vi "Model Calibration Control - 1D Table.vi"() -> ()   [LabVIEW 2011]
doc: "Sample numeric display item."
uses:
  <vilib>/NI Veristand/Display Template Support/Display Template Support.llb/cluster_Screen Item Settings.ctl
  <vilib>/NI Veristand/Display Template Support/Display Template Support.llb/cluster_Graph Scale Settings.ctl
  <vilib>/NI Veristand/Display Template Support/Display Template Support.llb/cluster_Graph Plot Settings.ctl
  NationalInstruments.VeriStand.SystemStorage
  Tables/TBL1D.xctl
  <vilib>/NI Veristand/Display Template Support/Display Template Support.llb/enum_Display Template Handler Minimal To Widget Msg.ctl
  <vilib>/NI Veristand/Display Template Support/Display Template Support.llb/enum_Display Template Handler Minimal To Workspace.ctl
  Tables/Limits TBL1D.ctl
  <vilib>/NI Veristand/Execution/Workspace/SystemState.ctl
  <vilib>/NI Veristand/Display Template Support/Display Template Support.llb/sub_Display Template Handler Custom.vi
  <vilib>/NI Veristand/Execution/ModelManager/NI VeriStand - Set Parameter 2D Array Values.vi
  <vilib>/NI Veristand/Execution/Workspace/NI VeriStand - Get Single Channel Value.vi
  <vilib>/NI Veristand/Execution/ModelManager/NI_VS ModelManager ExecutionAPI.lvlib
  <vilib>/NI Veristand/Execution/Workspace/NI_VS Workspace ExecutionAPI.lvlib
panel:
  in  "Paths":string[](array[string])
  out "Selected Parameter":string
  in  "TBL1D":cluster{"X":sgl[], "Y":sgl[]}(xcontrol)
  in  "NIVS.System Definition Root":refnum<k24>
  in  "Item.Data":T1
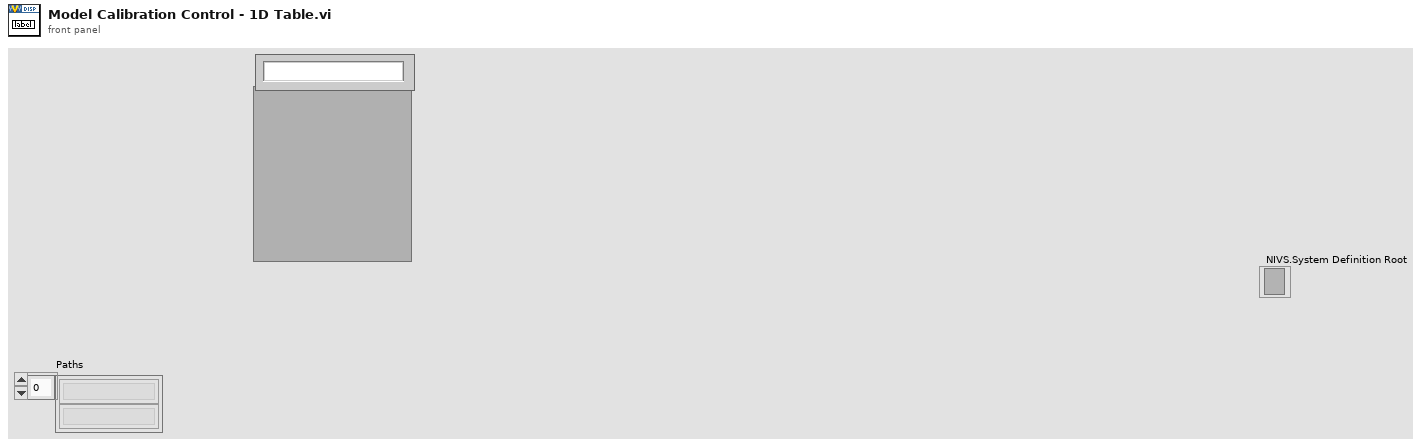
[diagram p1: front panel]
types:
  T1 = typedef "cluster_Screen Item Settings.ctl" = cluster{"Template VI":string, "Position X":i32, "Position Y":i32, "Custom":string, "Show Title Bar":bool, "ID":i32, "Always On Top":bool, "Allow Resize":bool, "Allow Minimize":bool, "Allow Close":bool, "Size to Screen":bool, "Screen.ID":i32, "State":enum16{"Normal", "New"}, "Title":string, "Window Bounds":cluster{"[0]":i16, "[1]":i16, "[2]":i16, "[3]":i16}, "Channel Ref":u64, "Unit":string, "Default Units?":bool, "Flash Limit?":bool, "Color 1":u32, "Color 2":u32, "Color 3":u32, "Color 4":u32, "Bck Color":u32, "Fore Color":u32, "Limit 1":dbl, "Limit 2":dbl, "Limit 3":dbl, "Limit 4":dbl, "Limit Mode 1":i32, "Limit Mode 2":i32, "Limit Mode 3":i32, "Limit Mode 4":i32, "Scale Precision":i32, "Scale Min":dbl, "Scale Max":dbl, "Format":i32, "Precision":i32, "Background Type":i32, "IDs":i32[], "Units":string[], "Labels":string[], "Scale Factor":dbl, "Scale Offset":dbl, "YScale Index":u32[], "XScale":T2, "YScales":T2[], "Plots":T3[], "Update Period":dbl, "History Length":dbl, "My.Ref":refnum<vi>, "Is Control?":bool, "Channel Paths":string[], "Custom Data":variant}
  T2 = typedef "cluster_Graph Scale Settings.ctl" = cluster{"Format":u8, "Precision":u8, "Fit":u8, "Label":string, "Use Default Label":bool, "Label Visible":bool, "Min":dbl, "Max":dbl}
  T3 = typedef "cluster_Graph Plot Settings.ctl" = cluster{"Bar Style":u8, "Fill To":i16, "Fill/PtColor":u32, "Line Style":u8, "Line Width":u8, "Color":u32, "Interp":u8, "Point Style":u8}
  T4 = typedef "TBL1D.xctl/Limits TBL1D.ctl" = cluster{"Min X":sgl, "Max X":sgl, "MaxDiff X":sgl, "MaxGrad X":sgl, "Min Y":sgl, "Max Y":sgl, "MaxDiff Y":sgl}
  T5 = typedef "enum_Display Template Handler Minimal To Workspace.ctl" = cluster{"Operation":enum16{"SetCustomData", "DeleteItem"}, "Data":variant}
  T6 = typedef "enum_Display Template Handler Minimal To Widget Msg.ctl" = enum16{"Stop", "LaunchConfigDialog"}
  T7 = typedef "NI_VS Workspace ExecutionAPI.lvlib/WorkspaceAPI.ctl" = refnum<k24>
  T8 = typedef "NI_VS ModelManager ExecutionAPI.lvlib/ModelManagerAPI.ctl" = refnum<k24>
  T9 = typedef "NI_VS Workspace ExecutionAPI.lvlib/SystemState.ctl" = u8
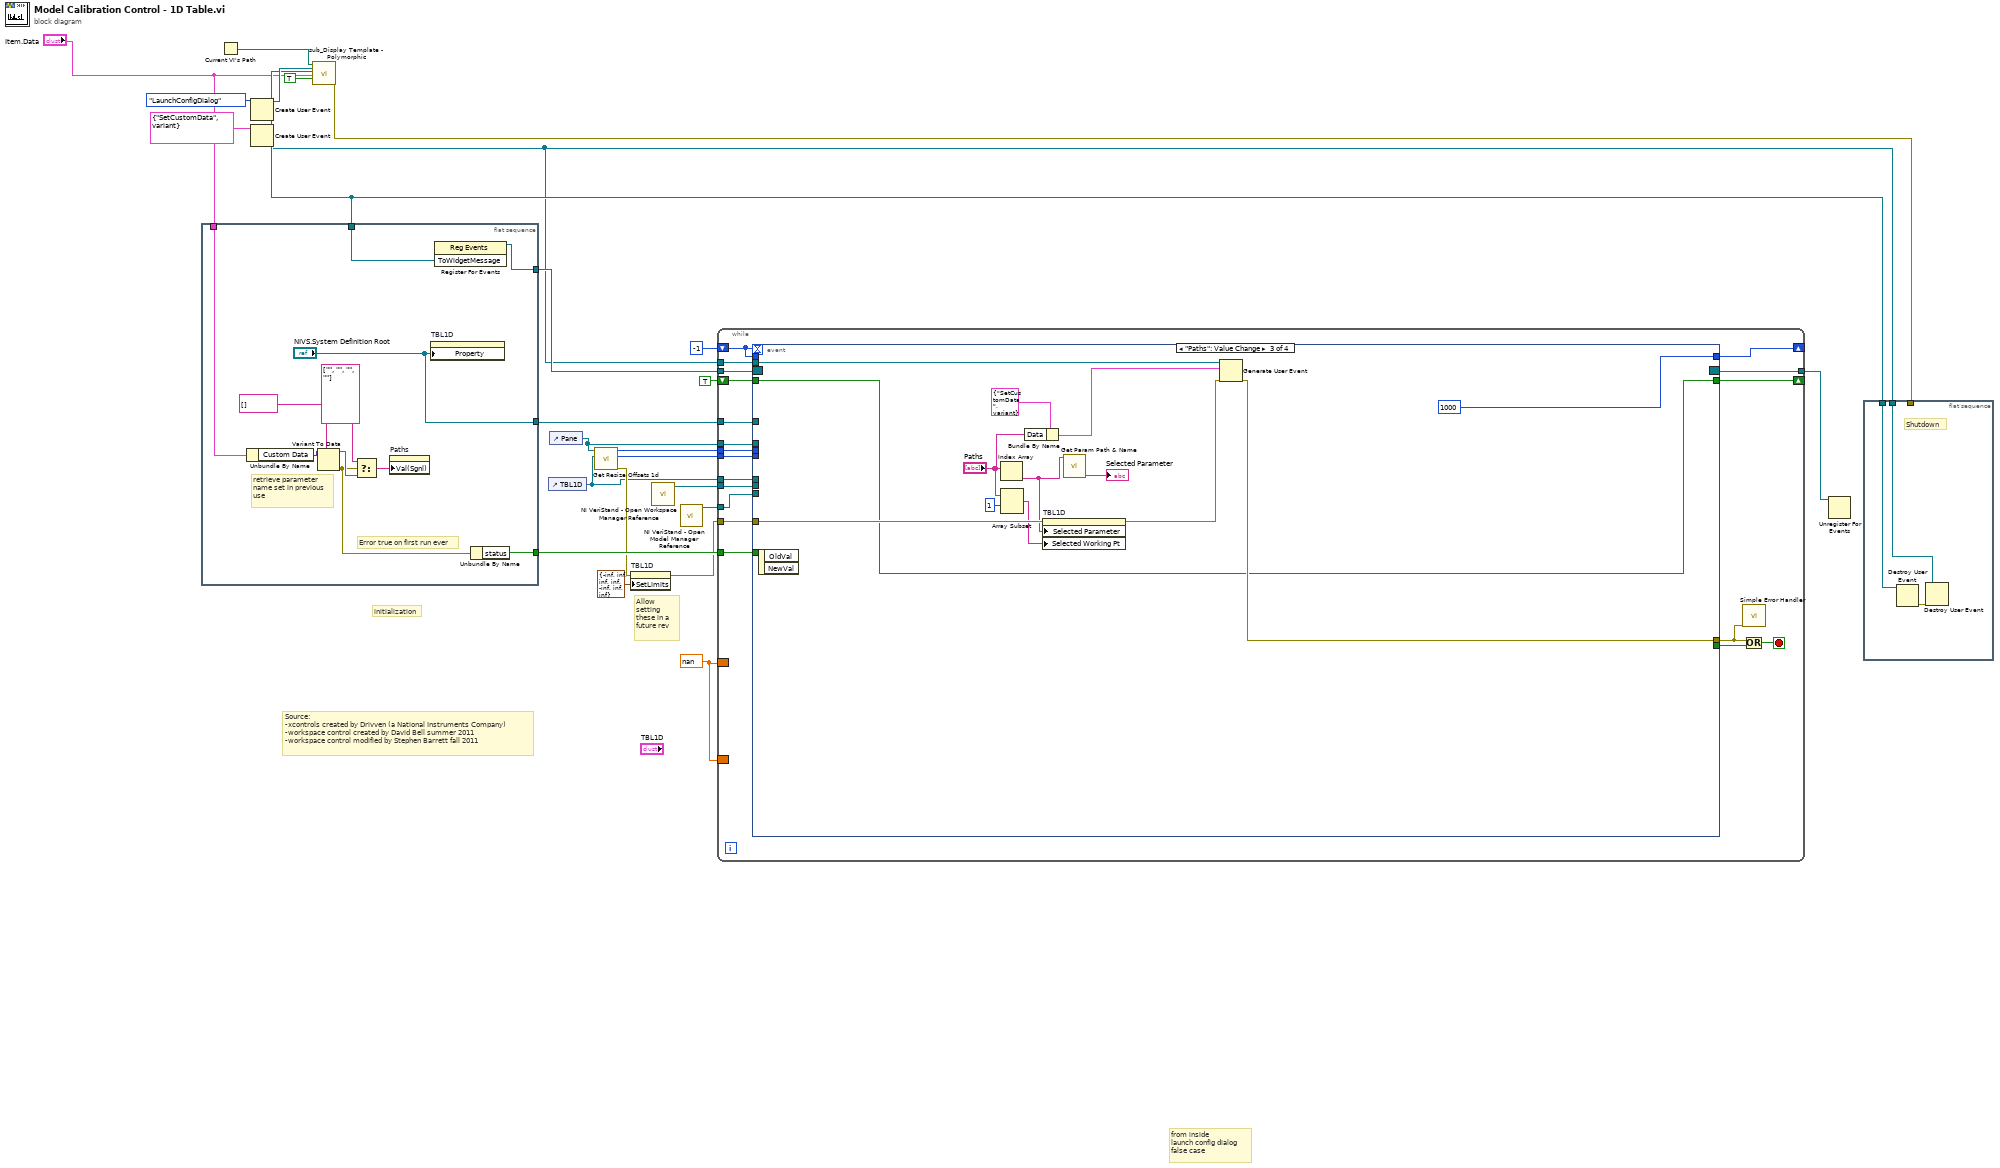
[diagram p0: block diagram]
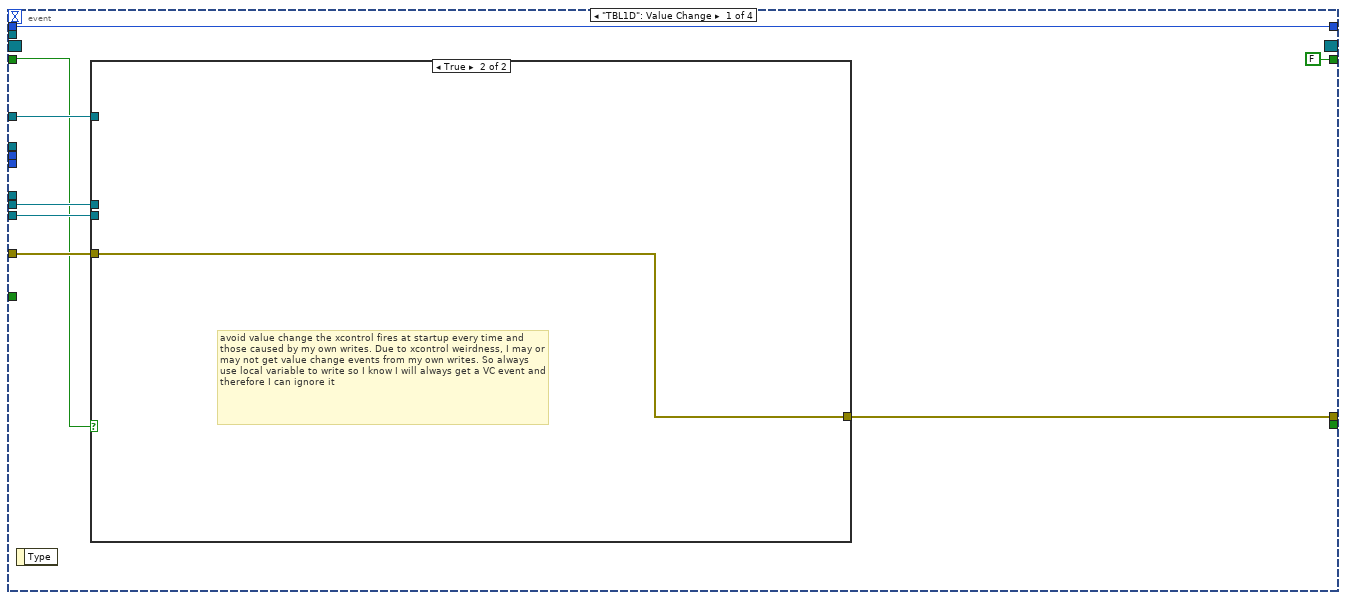
[diagram p2: hidden frame]
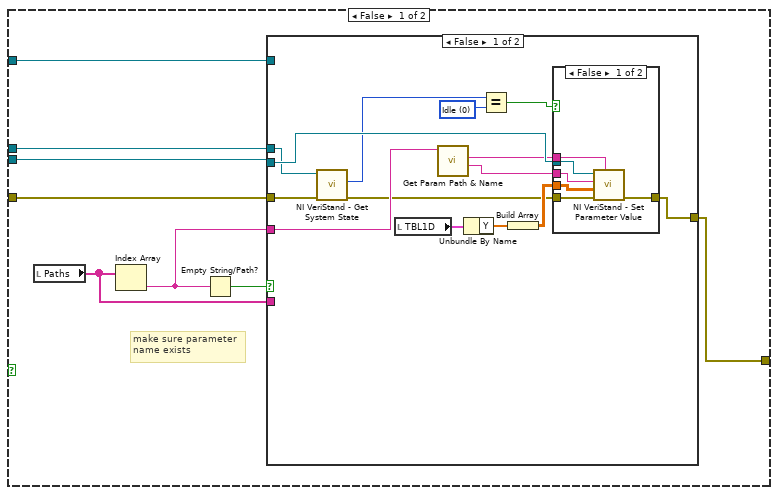
[diagram p3: hidden frame]
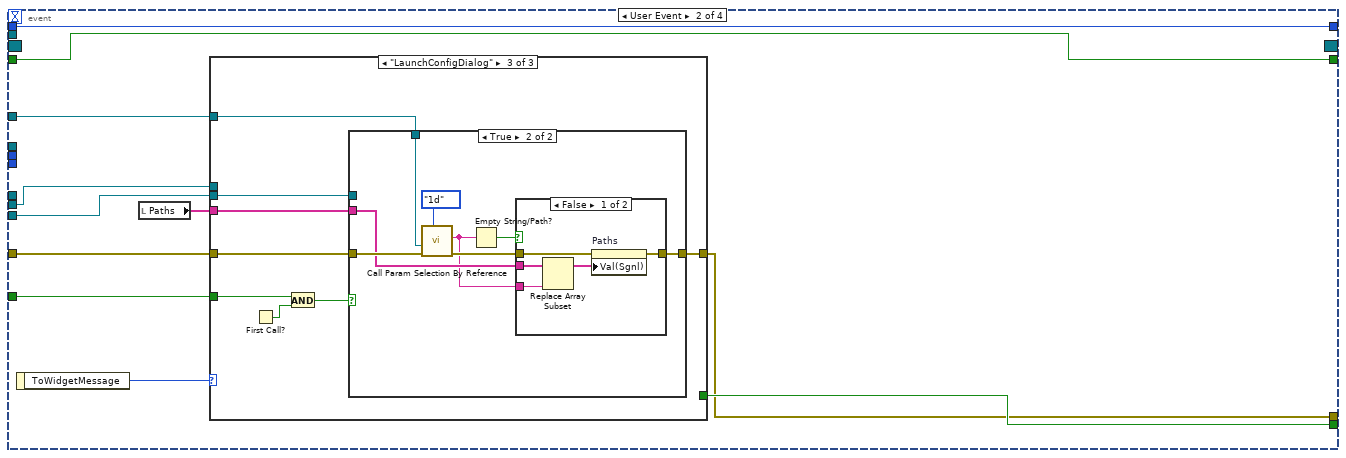
[diagram p6: hidden frame]
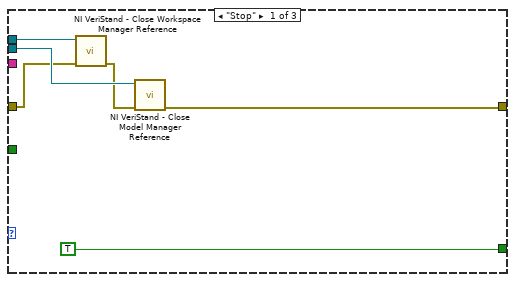
[diagram p7: hidden frame]
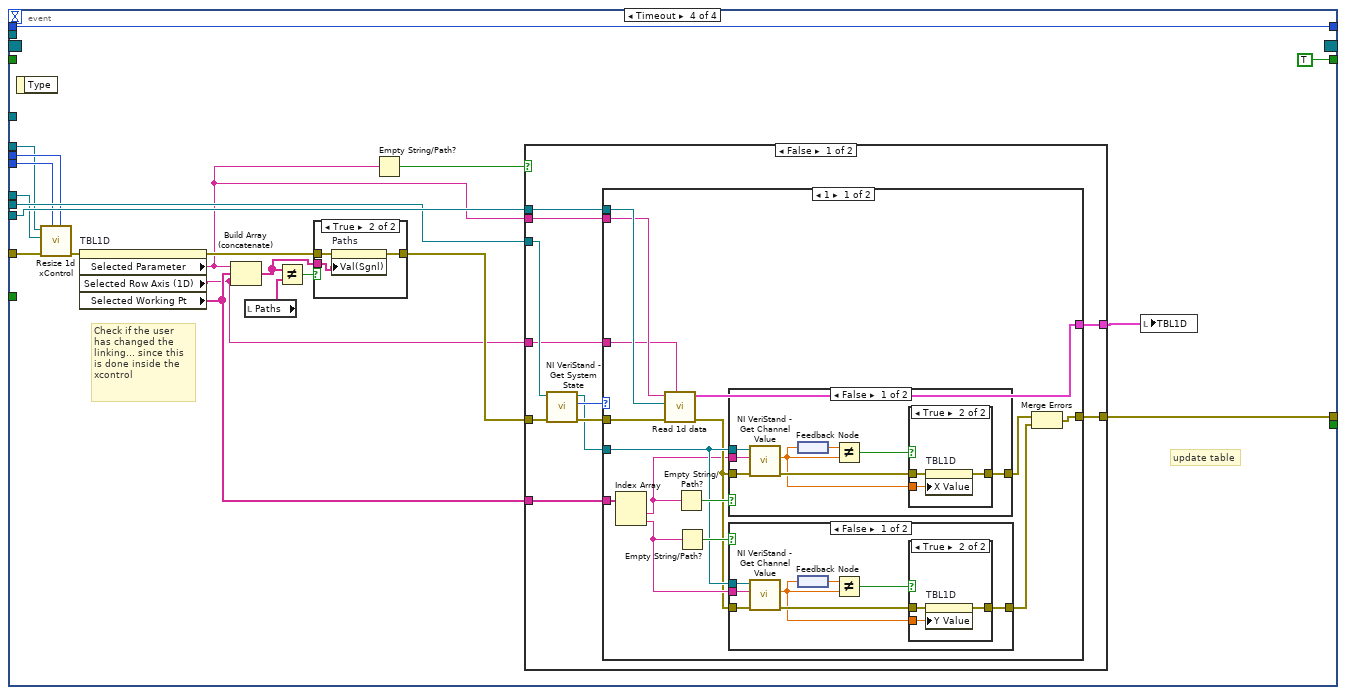
[diagram p11: hidden frame]
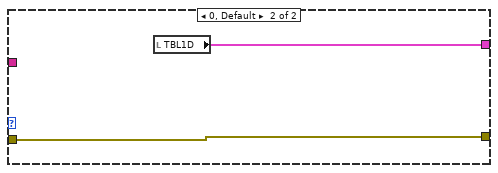
[diagram p17: hidden frame]
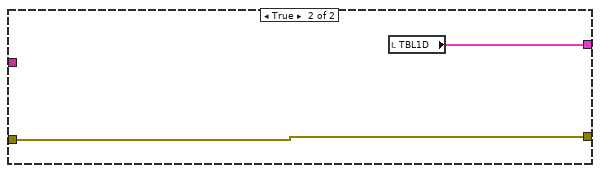
[diagram p18: hidden frame]
diagram:
  w3 = nan
  # "Source: \n-xcontrols created by Drivven (a National Instruments Company)\n-workspace control created by David Bell summer 2011\n-workspace control modified by Stephen Barrett fall 2011"
  # "Allow setting these in a future rev"
  # "initialization"
  # "from inside\nlaunch config dialog\nfalse case"
  n1 = flat-sequence {
    tunnel: [w35] -> w22
    tunnel: w20 -> [w34]
    tunnel: "Item.Data" -> [w32]
    tunnel: ["NIVS.System Definition Root"] -> w12
    tunnel: [w25] -> w11
    frame #0 {
      # "Error true on first run ever"
      # "retrieve parameter\nname set in previous\nuse"
      n2 = Unbundle By Name(w32) -> ("Custom Data"=w33:variant)
      n3 = Variant To Data(type=string[] [], Variant=w33) -> (data=w27:string[], error out=w26:errorcluster)  [unwired: 1 in]
      n4 = Select(t=string[] ["", "", "", ""], s=w26, f=w27) -> (s? t:f=w28:string[])
      n5 = property on="Paths" class="Arr (strict)"("Val(Sgnl)"=w28) -> ()  [unwired: 2 in, 2 out]
      n6 = property on="TBL1D" class="TBL1D (strict)"("Property"="NIVS.System Definition Root") -> ()  [unwired: 2 in, 2 out]
      n7 = register-events(w34) -> (reference out=w35:refnum<event-registration>)  [unwired: 2 in, 1 out]
      n8 = Unbundle By Name(w26) -> ("status"=w25:bool)
    }
  }
  n9 = Current VI's Path() -> (path=w18:path)
  n10 = Create User Event(user event datatype=enum_Display_Template_Handler_Minimal_To_Widget_Msg."LaunchConfigDialog" ("ToWidgetMessage")) -> (user event=w20:refnum<user-event>)  [unwired: 1 in, 1 out]
  n11 = Create User Event(user event datatype=T5 {"Operation"=enum."SetCustomData", "Data"=variant} ("Data")) -> (user event=w17:refnum<user-event>)  [unwired: 1 in, 1 out]
  n12 = call-poly <vilib>:"sub_Display Template - Polymorphic.vi"("Parent.Path"=w18, "ToWidgetEvent"=w20, "ToWorkspace"=w17, "Item.Data"="Item.Data", "Resizable"=TRUE) -> ("error out"=w24:errorcluster)  [unwired: 1 in, 13 out]
  n13 = control-ref of="TBL1D"() -> (w4:refnum<vi>)
  n14 = control-ref of="Pane"() -> (w5:refnum<vi>)
  n15 = call "Get Resize Offsets 1d.vi"("TBL1D Refnum"=w4, "Pane in"=w5) -> ("error out"=w8:errorcluster, "Width Offset"=w6:u32, "Height Offset"=w7:u32)  [unwired: 7 in]
  n16 = property on="TBL1D" class="TBL1D (strict)"(error in=w8, "SetLimits"=T4 {"Min X"=-inf, "Max X"=inf, "MaxDiff X"=inf, "MaxGrad X"=inf, "Min Y"=-inf, "Max Y"=inf, "MaxDiff Y"=inf}) -> (error out=w10:errorcluster)  [unwired: 1 in, 1 out]
  n17 = call <vilib>:"NI VeriStand - Open Workspace Manager Reference.vi"() -> ("WorkspaceManager"=w14:T7)  [unwired: 10 in, 1 out]
  n18 = call <vilib>:"NI VeriStand - Open Model Manager Reference.vi"() -> ("ModelManager"=w15:T8)  [unwired: 10 in, 1 out]
  n19 = while {
    tunnel: w22 -> [w54]
    tunnel: [w53] -> w21
    tunnel: w17 -> [w51]
    tunnel: w15 -> [w52]
    tunnel: w10 -> [w47]
    tunnel: w14 -> [w50]
    tunnel: w12 -> [w46]
    tunnel: w11 -> [w45]
    border: w3 -> [_]
    tunnel: w7 -> [w43]
    tunnel: w6 -> [w42]
    tunnel: w5 -> [w41]
    tunnel: w4 -> [w40]
    border: w3 -> [_]
    shift-right: [w38] -> _
    shift-left: -1 -> [w39]
    shift-right: [w36] -> _
    shift-left: TRUE -> [w37]
    stop <- w48 stop-if-true
    n20 = event shown="[2] \"Paths\": Value Change" {
      selector: w54 -> [_ _ _ _]
      dyn-events: [_ _ _ _] -> w53
      timeout: w39 -> [_ _ _ _]
      tunnel: w52 -> [w62 w103 _ w168]
      tunnel: w51 -> [_ _ w145 _]
      tunnel: [w60 w97 w142 w151] -> w44
      tunnel: [_ w104 _ _] -> w49
      tunnel: w50 -> [w61 w100 _ w167]
      tunnel: w47 -> [w59 w98 w144 w159]
      tunnel: w46 -> [w58 w101 _ _]
      tunnel: w45 -> [_ w96 _ _]
      tunnel: w43 -> [_ _ _ w156]
      tunnel: w42 -> [_ _ _ w157]
      tunnel: w41 -> [_ _ _ w155]
      tunnel: w40 -> [_ _ _ w154]
      tunnel: w39 -> [w57 w95 _ w150]
      tunnel: [w57 w95 1000 w150] -> w38
      tunnel: w37 -> [w56 w94 w135 _]
      tunnel: [FALSE w94 w135 TRUE] -> w36
      event "TBL1D": Value Change {
        n21 = event-data() -> ()  [unwired: 1 in, 1 out]
        n22 = case shown="True" w56 {
          tunnel: w62 -> [w70 _]
          tunnel: w61 -> [w69 _]
          tunnel: [w68 w93] -> w60
          tunnel: w59 -> [w67 w93]
          tunnel: w58 -> [w66 _]
          frame False {
            # "make sure parameter\nname exists"
            n23 = local read "Paths"() -> (w65:string[])
            n24 = Index Array(array=w65) -> (element=w63:string)  [unwired: 1 in]
            n25 = Empty String/Path?(string/path=w63) -> (empty?=w64:bool)
            n26 = case shown="False" w64 {
              tunnel: w70 -> [w83 _]
              tunnel: [w84 w92] -> w68
              tunnel: w69 -> [w80 _]
              tunnel: w67 -> [w75 w92]
              tunnel: w63 -> [w76 _]
              tunnel: w66 -> [_ _]
              tunnel: w65 -> [_ _]
              frame False {
                w78 = T9 0 items=["Idle", "Active"] ("System State")
                n27 = call <vilib>:"NI VeriStand - Get System State.vi"("error in (no error)"=w75, "WorkspaceManager in"=w80) -> ("error out"=w74:errorcluster, "System State"=w79:T9)  [unwired: 5 in, 3 out]
                n28 = local read "TBL1D"() -> (w77:cluster{"X":sgl[], "Y":sgl[]})
                n29 = call "Get Param Path & Name.vi"("Path"=w76) -> ("Parameter Path"=w73:string, "Controller name"=w72:string)  [unwired: 8 in, 1 out]
                n30 = Unbundle By Name(w77) -> ("Y"=w82:sgl[])
                n31 = Equal?(x=w79, y=w78) -> (x = y?=w71:bool)
                n32 = Build Array(w82) -> (w81:sgl[][])
                n33 = case shown="False" w71 {
                  tunnel: [w87 w91] -> w84
                  tunnel: w83 -> [w90 _]
                  tunnel: w81 -> [w89 _]
                  tunnel: w73 -> [w88 _]
                  tunnel: w74 -> [w86 w91]
                  tunnel: w72 -> [w85 _]
                  frame False {
                    n34 = call-poly <vilib>:"NI VeriStand - Set Parameter Value.vi"("Target"=w85, "error in (no error)"=w86, "Values"=w89, "Parameter"=w88, "ModelManager in"=w90) -> ("error out"=w87:errorcluster)  [unwired: 5 in, 1 out]
                  }
                  frame True {
                  }
                }
              }
              frame True {
              }
            }
          }
          frame True {
            # "avoid value change the xcontrol fires at startup every time and those caused by my own writes. Due to xcontrol weirdness, I may or may not get value change events from my own writes. So always use local variable to write so I know I will always get a VC event and therefore I can ignore it"
          }
        }
      }
      event User Event {
        n35 = event-data() -> ("ToWidgetMessage"=w102:T6)  [unwired: 1 in]
        n36 = local read "Paths"() -> (w99:string[])
        n37 = case shown="\"LaunchConfigDialog\"" w102 {
          tunnel: [TRUE ("1-D array?") _ _] -> w104
          tunnel: w103 -> [w108 _ w119]
          tunnel: w101 -> [_ _ w118]
          tunnel: w100 -> [w109 _ _]
          tunnel: w99 -> [_ _ w115]
          tunnel: w98 -> [w107 w111 w117]
          tunnel: [w105 w111 w116] -> w97
          tunnel: w96 -> [_ _ w114]
          frame "Stop" {
            n38 = call <vilib>:"NI VeriStand - Close Workspace Manager Reference.vi"("error in (no error)"=w107, "WorkspaceManager"=w109) -> ("error out"=w106:errorcluster)  [unwired: 9 in]
            n39 = call <vilib>:"NI VeriStand - Close Model Manager Reference.vi"("error in (no error)"=w106, "ModelManager"=w108) -> ("error out"=w105:errorcluster)  [unwired: 9 in]
          }
          frame Default {
          }
          frame "LaunchConfigDialog" {
            n40 = First Call?() -> (First Call?: T/F=w112:bool)
            n41 = And(x=w114, y=w112) -> (x .and. y?=w113:bool)
            n42 = case shown="True" w113 {
              tunnel: w119 -> [_ _]
              tunnel: w118 -> [_ w128]
              tunnel: w115 -> [_ w123]
              tunnel: w117 -> [w120 w127]
              tunnel: [w120 w124] -> w116
              frame False {
              }
              frame True {
                n43 = call "Call Param Selection By Reference.vi"("Param Size"=enum16{"Scalar", "1d", "2d"}."1d", "error in (no error)"=w127, "NIVS.System Definition Root"=w128) -> ("error out"=w125:errorcluster, "Selected NodePath"=w122:string)  [unwired: 7 in]
                n44 = Empty String/Path?(string/path=w122) -> (empty?=w121:bool)
                n45 = case shown="False" w121 {
                  tunnel: w125 -> [w133 w134]
                  tunnel: [w131 w134] -> w124
                  tunnel: w123 -> [w130 _]
                  tunnel: w122 -> [w129 _]
                  frame False {
                    n46 = Replace Array Subset(array=w130, new element=w129) -> (w132:string[])  [unwired: 1 in]
                    n47 = property on="Paths" class="Arr (strict)"(error in=w133, "Val(Sgnl)"=w132) -> (error out=w131:errorcluster)  [unwired: 1 in, 1 out]
                  }
                  frame True {
                  }
                }
              }
            }
          }
        }
      }
      event "Paths": Value Change {
        n48 = event-data() -> ()  [unwired: 1 in, 2 out]
        n49 = Index Array(array="Paths") -> (element=w141:string)  [unwired: 1 in]
        n50 = Array Subset(array="Paths", index=1) -> (w137:string[])  [unwired: 1 in]
        n51 = Bundle By Name(cluster=T5 {"Operation"=enum."SetCustomData", "Data"=variant} ("event data"), "Data"="Paths") -> (w147:T5)
        n52 = property on="TBL1D" class="TBL1D (strict)"(error in=w144, "Selected Parameter"=w141, "Selected Working Pt"=w137) -> (error out=w143:errorcluster)  [unwired: 1 in, 1 out]
        n53 = call "Get Param Path & Name.vi"("Path"=w141) -> ("Last Part"=→"Selected Parameter":string)  [unwired: 8 in, 2 out]
        n54 = Generate User Event(user event=w145, event data cluster=w147, error in=w143) -> (error out=w142:errorcluster)  [unwired: 1 out]
      }
      event Timeout {
        # "Check if the user has changed the linking... since this is done inside the xcontrol"
        # "update table"
        n55 = event-data() -> ()  [unwired: 1 in, 1 out]
        n56 = call "Resize 1d xControl.vi"("Height Offset"=w156, "Width Offset"=w157, "error in (no error)"=w159, "Control in"=w154, "Pane"=w155) -> ("error out"=w158:errorcluster)  [unwired: 6 in]
        n57 = property on="TBL1D" class="TBL1D (strict)"(error in=w158) -> (error out=w164:errorcluster, "Selected Parameter"=w160:string, "Selected Row Axis (1D)"=w152:string, "Selected Working Pt"=w153:string[])  [unwired: 1 in, 1 out]
        n58 = Build Array (concatenate)(w160, w153, w152) -> (w161:string[])
        n59 = local read "Paths"() -> (w165:string[])
        n60 = Not Equal?(x=w161, y=w165) -> (x != y?=w162:bool)
        n61 = case shown="True" w162 {
          tunnel: w164 -> [w169 w172]
          tunnel: [w169 w171] -> w163
          tunnel: w161 -> [_ w170]
          frame False {
          }
          frame True {
            n62 = property on="Paths" class="Arr (strict)"(error in=w172, "Val(Sgnl)"=w170) -> (error out=w171:errorcluster)  [unwired: 1 in, 1 out]
          }
        }
        n63 = Empty String/Path?(string/path=w160) -> (empty?=w166:bool)
        n64 = case shown="False" w166 {
          tunnel: [w183 w227] -> w148
          tunnel: [w182 w228] -> w151
          tunnel: w160 -> [w174 _]
          tunnel: w168 -> [w181 _]
          tunnel: w167 -> [w180 _]
          tunnel: w163 -> [w179 w228]
          tunnel: w153 -> [w177 _]
          tunnel: w152 -> [w173 _]
          frame False {
            n65 = call <vilib>:"NI VeriStand - Get System State.vi"("error in (no error)"=w179, "WorkspaceManager in"=w180) -> ("error out"=w178:errorcluster, "System State"=w176:T9, "WorkspaceManager  out"=w175:T7)  [unwired: 5 in, 2 out]
            n66 = case shown="1" w176 {
              tunnel: [w196 w225] -> w183
              tunnel: [w188 w226] -> w182
              tunnel: w181 -> [w198 _]
              tunnel: w178 -> [w197 w226]
              tunnel: w177 -> [w194 _]
              tunnel: w175 -> [w190 _]
              tunnel: w174 -> [w185 _]
              tunnel: w173 -> [w184 _]
              frame 1 {
                n67 = Index Array(array=w194) -> (element #1=w186:string, element #2=w191:string)  [unwired: 2 in]
                n68 = call "Read 1d data.vi"("Row Axis Path"=w184, "error in (no error)"=w197, "ModelManager"=w198, "Parameter Path"=w185) -> ("error out"=w189:errorcluster, "TBL1D"=w196:cluster{"X":sgl[], "Y":sgl[]})  [unwired: 6 in]
                n69 = Empty String/Path?(string/path=w186) -> (empty?=w195:bool)
                n70 = Empty String/Path?(string/path=w191) -> (empty?=w192:bool)
                n71 = case shown="False" w195 {
                  tunnel: w190 -> [w219 _]
                  tunnel: w186 -> [w218 _]
                  tunnel: w189 -> [w217 w224]
                  tunnel: [w214 w224] -> w193
                  frame False {
                    n72 = call-poly <vilib>:"NI VeriStand - Get Channel Value.vi"("error in (no error)"=w217, "Channel"=w218, "WorkspaceManager in"=w219) -> ("error out"=w215:errorcluster, "Value"=w213:dbl)  [unwired: 6 in, 1 out]
                    n73 = feedback-in #1(w213) -> ()
                    n74 = feedback #1() -> (w216:dbl)
                    n75 = Not Equal?(x=w216, y=w213) -> (x != y?=w212:bool)
                    n76 = case shown="True" w212 {
                      tunnel: w215 -> [w220 w223]
                      tunnel: [w220 w222] -> w214
                      tunnel: w213 -> [_ w221]
                      frame False {
                      }
                      frame True {
                        n77 = property on="TBL1D" class="TBL1D (strict)"(error in=w223, "X Value"=w221) -> (error out=w222:errorcluster)  [unwired: 1 in, 1 out]
                      }
                    }
                  }
                  frame True {
                  }
                }
                n78 = case shown="False" w192 {
                  tunnel: w190 -> [w206 _]
                  tunnel: w191 -> [w205 _]
                  tunnel: w189 -> [w204 w211]
                  tunnel: [w201 w211] -> w187
                  frame False {
                    n79 = call-poly <vilib>:"NI VeriStand - Get Channel Value.vi"("error in (no error)"=w204, "Channel"=w205, "WorkspaceManager in"=w206) -> ("error out"=w202:errorcluster, "Value"=w200:dbl)  [unwired: 6 in, 1 out]
                    n80 = feedback-in #2(w200) -> ()
                    n81 = feedback #2() -> (w203:dbl)
                    n82 = Not Equal?(x=w203, y=w200) -> (x != y?=w199:bool)
                    n83 = case shown="True" w199 {
                      tunnel: w202 -> [w207 w210]
                      tunnel: [w207 w209] -> w201
                      tunnel: w200 -> [_ w208]
                      frame False {
                      }
                      frame True {
                        n84 = property on="TBL1D" class="TBL1D (strict)"(error in=w210, "Y Value"=w208) -> (error out=w209:errorcluster)  [unwired: 1 in, 1 out]
                      }
                    }
                  }
                  frame True {
                  }
                }
                n85 = Merge Errors(w193, w187) -> (w188:errorcluster)
              }
              frame 0, Default {
                n86 = local read "TBL1D"() -> (w225:cluster{"X":sgl[], "Y":sgl[]})
              }
            }
          }
          frame True {
            n87 = local read "TBL1D"() -> (w227:cluster{"X":sgl[], "Y":sgl[]})
          }
        }
        n88 = local write "TBL1D"(w148) -> ()
      }
    }
    n89 = call <vilib>:"Simple Error Handler.vi"("error in (no error)"=w44) -> ()  [unwired: 4 in, 5 out]
    n90 = Or(x=w44, y=w49) -> (x .or. y?=w48:bool)
  }
  n91 = Unregister For Events(event registration refnum=w21) -> ()  [unwired: 1 in, 1 out]
  n92 = flat-sequence {
    tunnel: w24 -> [_]
    tunnel: w20 -> [w231]
    tunnel: w17 -> [w230]
    frame #0 {
      # "Shutdown"
      n93 = Destroy User Event(user event=w231) -> (error out=w229:errorcluster)  [unwired: 1 in]
      n94 = Destroy User Event(user event=w230, error in=w229) -> ()  [unwired: 1 out]
    }
  }
